vi "Main Page.vi"(8 "error in (no error)":errorcluster, 11 "Node Ptr":T1 format="%.0x") -> (0 "error out":errorcluster)   [LabVIEW 2016, in "FPGA RM Test Client System Explorer.lvlib"]
uses:
  FPGA RM Test Client System Explorer.lvlib
  <vilib>/NI Veristand/Custom Device API/Custom Device Item Ref.ctl
  <vilib>/NI VeriStand/Custom Device API/Custom Device API.lvlib
  Source/FPGA Resource Manager.lvlib
  Source/Filters/RIO Device Filter/RIO Device Filter.lvclass
  Source/Filters/Input Type Filter/Input Type Filter.lvclass
  Source/Filters/AND Filter/AND Filter.lvclass
panel:
  in  "Available FPGA resources":string(tree)
  out "Version":string
  in  "Specific Header":cluster{"Section Name":string}={"Section Name"="Custom Device Item Settings"}
  in  "General Header":cluster{"Section Name":string}={"Section Name"="General Custom Device Settings"}
  in  "Description":string
  in  "Name":string
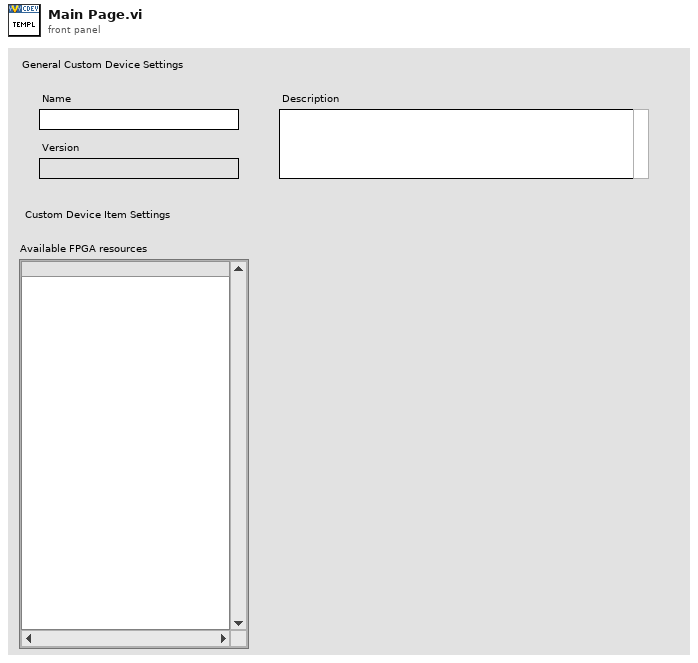
[diagram p1: front panel]
types:
  T1 = typedef "Custom Device API.lvlib/Custom Device Item Ref.ctl" = u64
  T2 = enum16{"Scalar Inputs", "Scalar Outputs", "Waveform Inputs", "Waveform Outputs"}
  T3 = typedef "Custom Device API.lvlib/Custom Device Item Info.ctl" = cluster{"Name":string, "Is Channel":bool, "GUID":string, "Is Waveform":bool}
  T4 = typedef "Custom Device API.lvlib/Custom Device Commands.ctl" = enum16{"Default", "Item renamed", "Shutdown", "Dynamic button pressed"}
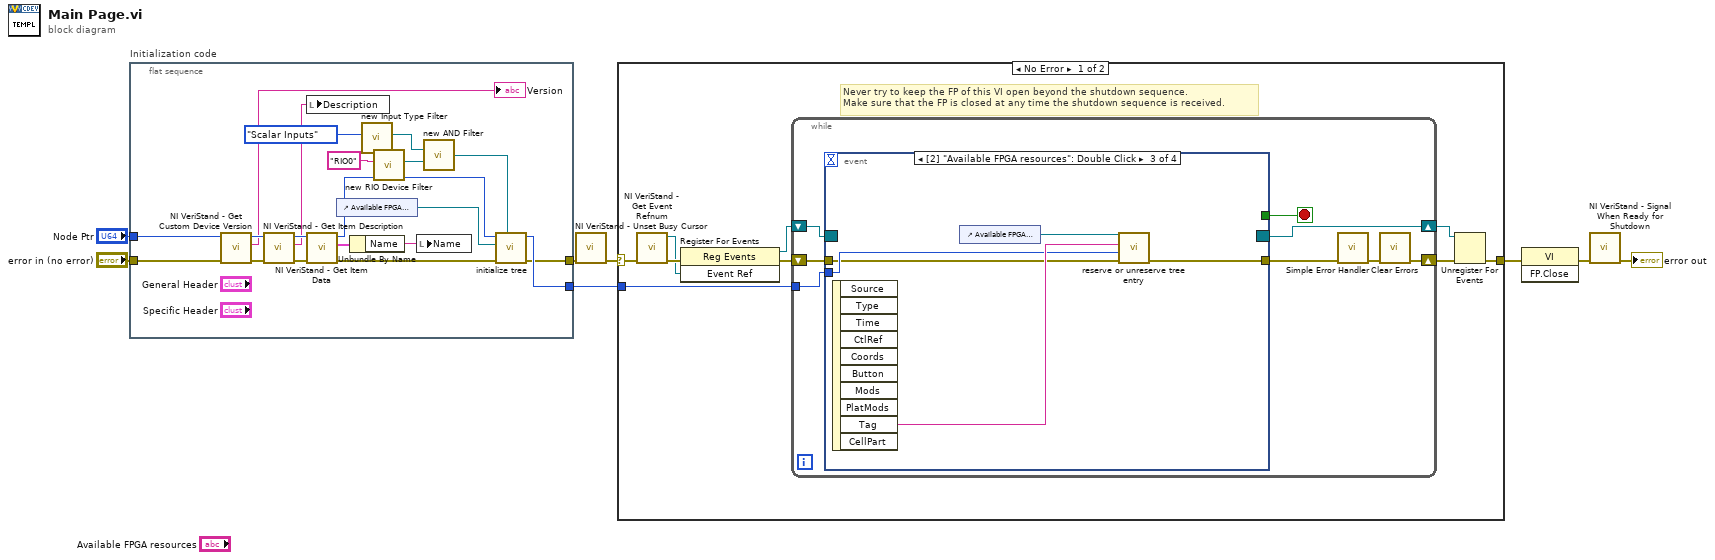
[diagram p0: block diagram]
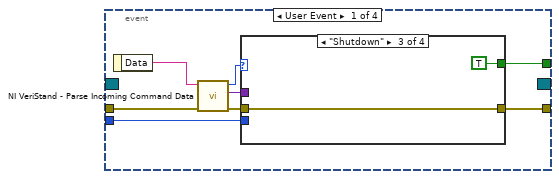
[diagram p2: hidden frame]
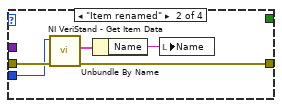
[diagram p4: hidden frame]
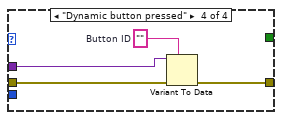
[diagram p5: hidden frame]
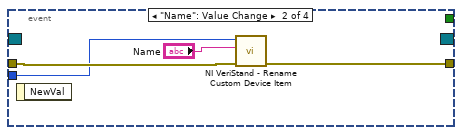
[diagram p6: hidden frame]
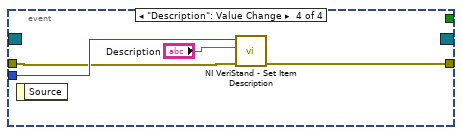
[diagram p7: hidden frame]
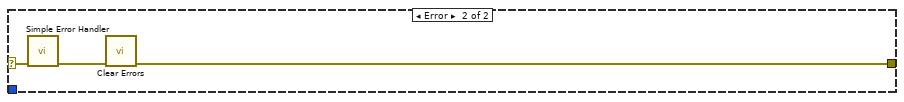
[diagram p8: hidden frame]
diagram:
  n1 = flat-sequence "Initialization code" {
    tunnel: "error in (no error)" -> [w21]
    tunnel: "Node Ptr" -> [w25]
    tunnel: [w15] -> w5
    tunnel: [w16] -> w2
    frame #0 {
      n2 = call <vilib>:"NI VeriStand - Get Custom Device Version.vi"("error in (no error)"=w21, "Device Ref in"=w25) -> ("error out"=w24:errorcluster, "Value"=→"Version":string, "Device Ref out"=w23:T1)  [unwired: 7 in]
      n3 = call <vilib>:"NI VeriStand - Get Item Description.vi"("error in (no error)"=w24, "Item Ref in"=w23) -> ("error out"=w27:errorcluster, "Description"=w19:string, "Item Ref out"=w28:T1)  [unwired: 7 out]
      n4 = local write "Description"(w19) -> ()
      n5 = call <vilib>:"NI VeriStand - Get Item Data.vi"("error in (no error)"=w27, "Item Ref in"=w28) -> ("error out"=w18:errorcluster, "Item Info"=w26:T3, "Item Ref out"=w17:T1)  [unwired: 7 out]
      n6 = control-ref of="Available FPGA resources"() -> (w14:refnum<vi>)
      n7 = Unbundle By Name(w26) -> ("Name"=w20:string)
      n8 = call "new Input Type Filter.vi"("Input Type"=T2."Scalar Inputs") -> ("input type filter out"=w12:refnum<class "Filter.lvclass">)  [unwired: 10 in]
      n9 = call "new RIO Device Filter.vi"("RIO Device Name"="RIO0") -> ("RIO device filter out"=w11:refnum<class "Filter.lvclass">)  [unwired: 9 in]
      n10 = local write "Name"(w20) -> ()
      n11 = call "new AND Filter.vi"("a"=w12, "b"=w11) -> ("a and b"=w10:refnum<class "Filter.lvclass">)  [unwired: 13 in]
      n12 = call "initialize tree.vi"("Filter in"=w10, "error in (no error)"=w18, "TreeControl in"=w14, "Node Ptr"=w17) -> ("error out"=w15:errorcluster, "Item Ref out"=w16:T1)  [unwired: 6 in]
    }
  }
  n13 = call <vilib>:"NI VeriStand - Unset Busy Cursor.vi"("error in (no error)"=w5) -> ("error out"=w4:errorcluster)  [unwired: 10 out]
  n14 = case shown="No Error" w4 {
    selector: w4 -> [w29 w81]
    tunnel: [w34 w79] -> w8
    tunnel: w2 -> [w30 _]
    frame No Error {
      # "Never try to keep the FP of this VI open beyond the shutdown sequence.\nMake sure that the FP is closed at any time the shutdown sequence is received."
      n15 = call <vilib>:"NI VeriStand - Get Event Refnum.vi"("error in (no error)"=w29) -> ("error out"=w37:errorcluster, "Event Ref"=w33:refnum<user-event>)  [unwired: 9 out]
      n16 = register-events(error in=w37, w33) -> (reference out=w31:refnum<event-registration>, error out=w32:errorcluster)  [unwired: 1 in]
      n17 = while {
        tunnel: w30 -> [w41]
        shift-right: [w38] -> w35
        shift-left: w32 -> [w44]
        shift-right: [w45] -> w36
        shift-left: w31 -> [w43]
        stop <- w42 stop-if-true
        n18 = event shown="[2] \"Available FPGA resources\": Double Click" {
          selector: w43 -> [_ _ _ _]
          dyn-events: [_ _ _ _] -> w45
          timeout: _ -> [_ _ _ _]
          tunnel: w44 -> [w53 w69 w71 w77]
          tunnel: [w49 _ _ _] -> w42
          tunnel: [w48 w68 w70 w76] -> w40
          tunnel: w41 -> [w47 w67 w72 w78]
          event User Event {
            n19 = event-data() -> ("Data"=w52:string)  [unwired: 1 out]
            n20 = call <vilib>:"NI VeriStand - Parse Incoming Command Data.vi"("error in (no error)"=w53, "Incoming data"=w52) -> ("error out"=w51:errorcluster, "Outgoing data"=w46:variant, "Action"=w50:T4)  [unwired: 7 out]
            n21 = case shown="\"Shutdown\"" w50 {
              tunnel: w51 -> [w54 w59 w60 w65]
              tunnel: [_ _ TRUE _] -> w49
              tunnel: [w54 w56 w60 w62] -> w48
              tunnel: w47 -> [_ w58 _ _]
              tunnel: w46 -> [_ _ _ w64]
              frame "Default", Default {
              }
              frame "Item renamed" {
                n22 = call <vilib>:"NI VeriStand - Get Item Data.vi"("error in (no error)"=w59, "Item Ref in"=w58) -> ("error out"=w56:errorcluster, "Item Info"=w57:T3)  [unwired: 8 out]
                n23 = Unbundle By Name(w57) -> ("Name"=w55:string)
                n24 = local write "Name"(w55) -> ()
              }
              frame "Shutdown" {
              }
              frame "Dynamic button pressed" {
                w63 = ""  # Button ID
                n25 = Variant To Data(error in=w65, type=w63, Variant=w64) -> (error out=w62:errorcluster)  [unwired: 1 out]
              }
            }
          }
          event "Name": Value Change {
            n26 = event-data() -> ()  [unwired: 2 out]
            n27 = call <vilib>:"NI VeriStand - Rename Custom Device Item.vi"("error in (no error)"=w69, "New Name"="Name", "Item Ref in"=w67) -> ("error out"=w68:errorcluster)  [unwired: 1 in, 7 out]
          }
          event "Available FPGA resources": Double Click {
            n28 = event-data() -> ("Tag"=w73:string)  [unwired: 10 out]
            n29 = control-ref of="Available FPGA Resources"() -> (w74:refnum<vi>)
            n30 = call "reserve or unreserve tree entry.vi"("error in (no error)"=w71, "Item Ref in"=w72, "Tag"=w73, "TreeControl in"=w74) -> ("error out"=w70:errorcluster)  [unwired: 7 in]
          }
          event "Description": Value Change {
            n31 = event-data() -> ()  [unwired: 2 out]
            n32 = call <vilib>:"NI VeriStand - Set Item Description.vi"("error in (no error)"=w77, "Description"="Description", "Item Ref in"=w78) -> ("error out"=w76:errorcluster)  [unwired: 8 out]
          }
        }
        n33 = call <vilib>:"Simple Error Handler.vi"("error in (no error)"=w40) -> ("error out"=w39:errorcluster)  [unwired: 1 in, 7 out]
        n34 = call <vilib>:"Clear Errors.vi"("error in (no error)"=w39) -> ("error out"=w38:errorcluster)  [unwired: 1 in, 5 out]
      }
      n35 = Unregister For Events(event registration refnum=w36, error in=w35) -> (error out=w34:errorcluster)
    }
    frame Error {
      n36 = call <vilib>:"Simple Error Handler.vi"("error in (no error)"=w81) -> ("error out"=w80:errorcluster)  [unwired: 1 in, 7 out]
      n37 = call <vilib>:"Clear Errors.vi"("error in (no error)"=w80) -> ("error out"=w79:errorcluster)  [unwired: 1 in, 5 out]
    }
  }
  n38 = invoke class="VI" method="FP.Close"(error in=w8) -> (error out=w7:errorcluster)  [unwired: 2 in, 2 out]
  n39 = call <vilib>:"NI VeriStand - Signal When Ready for Shutdown.vi"("error in (no error)"=w7) -> ("error out"=→"error out":errorcluster)  [unwired: 10 out]
